vi "Async VI Control_Get VI Names.vi"(8 "error in":errorcluster, 11 "VI References":refnum<vi>[](array[refnum])) -> (0 "error out":errorcluster, 3 "Clone Names":string[](array[string]))   [LabVIEW 2013, in "CANOpen Addon Custom Device.lvlib"]
uses:
  CANOpen Addon Custom Device.lvlib
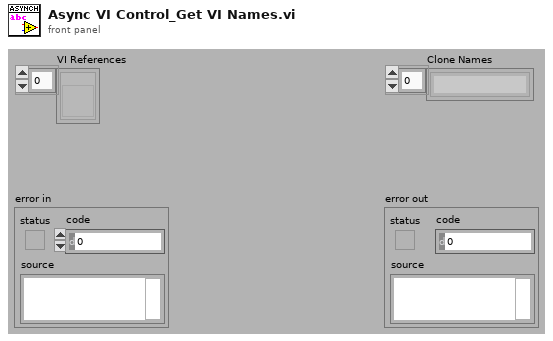
[diagram p1: front panel]
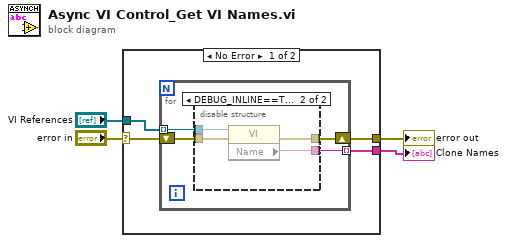
[diagram p0: block diagram]
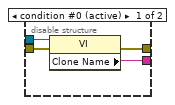
[diagram p2: hidden frame]
diagram:
  n1 = case shown="No Error" "error in" {
    selector: "error in" -> [w5 w21]
    tunnel: "VI References" -> [w8 _]
    tunnel: [w7 _] -> w1
    tunnel: [w6 w21] -> w3
    frame No Error {
      n2 = for {
        tunnel: w8 -> [w12] mode=indexing
        tunnel: [w11] -> w7 mode=indexing
        shift-right: [w10] -> w6
        shift-left: w5 -> [w9]
        n3 = disable-structure shown="DEBUG_INLINE==TRUE" {
          disable-tunnel: w12 -> [w16 w20]
          disable-tunnel: [w15 w19] -> w11
          disable-tunnel: [w14 w18] -> w10
          disable-tunnel: w9 -> [w13 w17]
          frame condition #0 (active) {
            n4 = property class="VI"(reference=w16, error in=w13) -> (error out=w14:errorcluster, "Clone Name"=w15:string)  [unwired: 1 out]
          }
          frame condition #1 {
            n5 = property class="VI"(reference=w20, error in=w17) -> (error out=w18:errorcluster, "Name"=w19:string)  [unwired: 1 out]
          }
        }
      }
    }
    frame Error {
    }
  }
  "error out" <- w3
  "Clone Names" <- w1
